vi "WFComposeCan.vi"   [LabVIEW 2013]
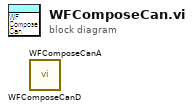
[diagram p0: block diagram]
diagram:
  n1 = call "WFComposeCanD.vi"() -> ()  [unwired: 10 in, 2 out]
  n2 = call "WFComposeCanA.vi"() -> ()  [unwired: 10 in, 2 out]
